vi "refMgr_Example5.vi"() -> ()   [LabVIEW 2017]
uses:
  40be52e9-3771-4604-be95-a9dd39ca470b.vi
  <userlib>/_NEVSTOP/TagDB/_Support/DataAccess/data-Write.vi
  <userlib>/_NEVSTOP/TagDB/_Support/DataAccess/_NameCacher.vi
  <userlib>/_NEVSTOP/TagDB/_Support/DataAccess/_datatypeChecker.vi
  <userlib>/_NEVSTOP/TagDB/_Support/DataAccess/TagDB Ref to DVR.vi
  <vilib>/Utility/Data Type/Get Type Information.vi
  <vilib>/Utility/error.llb/Trim Whitespace.vi
  <userlib>/_NEVSTOP/TagDB/_Support/Error/_[error50000]Invalid DB REF.vi
  RefManager/_Support/UISync/_Pull Controls Value to DPs(Refmgr).vi
  RefManager/_Support/UISync/_Publish DP Indicators(Refmgr).vi
  RefManager/TagDB RefManager.lvlib
  <userlib>/_NEVSTOP/TagDB/TagDB.lvlib
panel:
  out "Numeric 6":dbl
  in  "Numeric 5":dbl
  out "Numeric 1":dbl
  in  "Numeric 0":dbl
  in  "Tab Control":enum32{"Page 1", "Page 2"}(tab)
  out "Numeric 3":dbl
  out "Numeric 4":dbl
  out "Numeric 8":dbl
  out "Numeric 9":dbl
  in  "Numeric 7":dbl
  in  "Numeric 2":dbl
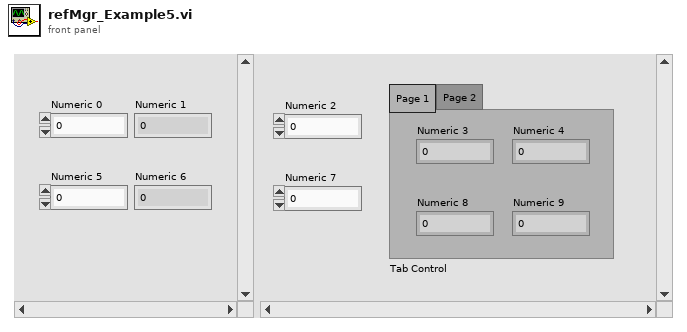
[diagram p1: front panel]
types:
  T1 = typedef "TagDB.lvlib/TagDB.ctl" = refnum<k1>
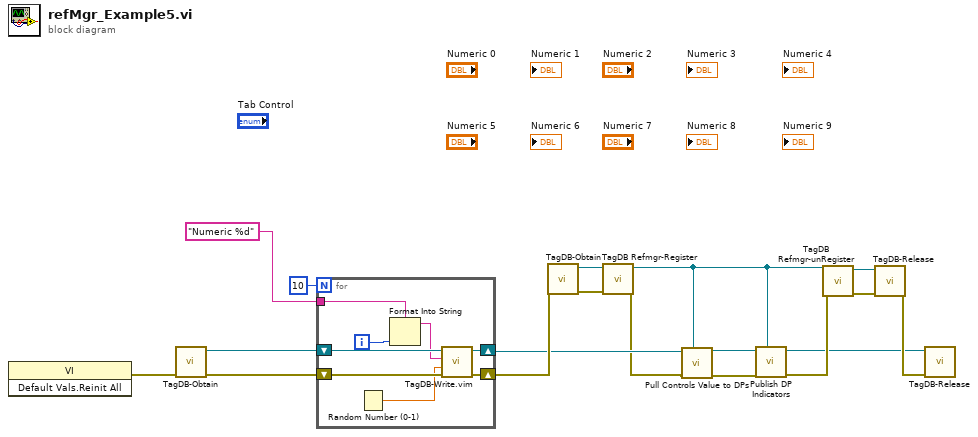
[diagram p0: block diagram]
diagram:
  n1 = invoke class="VI" method="Default Vals.Reinit All"() -> (error out=w11:errorcluster)  [unwired: 3 in, 2 out]
  n2 = call <userlib>:"TagDB-Obtain.vi"("error in (no error)"=w11) -> ("error out"=w9:errorcluster, "TagDB"=w16:T1)  [unwired: 4 in, 1 out]
  n3 = for {
    N: 10 -> [_]
    tunnel: "Numeric %d" ("name") -> [w22]
    shift-right: [w25] -> w5
    shift-left: w16 -> [w26]
    shift-right: [w19] -> w7
    shift-left: w9 -> [w24]
    i -> [w20]
    n4 = Random Number (0-1)() -> (number: 0 to 1=w21:dbl)
    n5 = Format Into String(format string=w22, w20) -> (resulting string=w23:string)  [unwired: 2 in, 1 out]
    n6 = call "TagDB-Write.vim"("error in (no error)"=w24, "Value"=w21, "name"=w23, "TagDB"=w26) -> ("error out"=w19:errorcluster, "TagDB(dup)"=w25:T1)  [unwired: 5 in, 1 out]
  }
  n7 = call <userlib>:"TagDB-Obtain.vi"("error in (no error)"=w7) -> ("error out"=w17:errorcluster, "TagDB"=w18:T1)  [unwired: 4 in, 1 out]
  n8 = call "TagDB Refmgr-Register.vi"("error in (no error)"=w17, "TagDB in"=w18) -> ("error out"=w4:errorcluster, "TagDB out"=w1:T1)  [unwired: 7 in, 1 out]
  n9 = call-poly "Pull Controls Value to DPs.vi"("VIRef(Caller VI)"=w1, "error in (no error)"=w4, "SILAPI In"=w5) -> ("error out"=w3:errorcluster, "SILAPI Out"=w2:T1)  [unwired: 6 in, 1 out]
  n10 = call-poly "Publish DP Indicators.vi"("VIRef(Caller VI)"=w1, "error in (no error)"=w3, "SILAPI In"=w2) -> ("error out"=w13:errorcluster, "SILAPI Out"=w8:T1)  [unwired: 6 in, 1 out]
  n11 = call "TagDB Refmgr-unRegister.vi"("error in (no error)"=w13, "TagDB in"=w1) -> ("error out"=w15:errorcluster, "TagDB out"=w14:T1)  [unwired: 8 in]
  n12 = call <userlib>:"TagDB-Release.vi"("error in (no error)"=w15, "TagDB"=w14) -> ("error out"=w12:errorcluster)  [unwired: 9 in]
  n13 = call <userlib>:"TagDB-Release.vi"("error in (no error)"=w12, "TagDB"=w8) -> ()  [unwired: 9 in, 1 out]
